vi "OrderDeviceList.vi"(8 "error in (no error)":errorcluster, 11 "Device List In":refnum<class "Device.lvclass">[](array[class])) -> (0 "error out":errorcluster, 2 "Changes Made":bool, 3 "Device List Out":refnum<class "Device.lvclass">[](array[class]))   [LabVIEW 2013]
uses:
  DeviceVIs/Device/Device.lvclass
  DeviceVIs/Pulseblaster/Pulseblaster.lvclass
  ColumnVIs/Column/Column.lvclass
  ColumnVIs/ModeCol/ModeCol.lvclass
  ColumnVIs/GroupCol/GroupCol.lvclass
  ColumnVIs/DigitalCol/DigitalCol.lvclass
  ColumnVIs/TriggerCol/TriggerCol.lvclass
  DeviceVIs/NI Card/NI Card.lvclass
  DeviceVIs/Slave_Pulseblaster/Slave_Pulseblaster.lvclass
panel:
  in  "Cancel Button":bool
  in  "OK Button":bool
  out "Master Name":string="Master Device"
  in  "Device Order":i32(listbox)
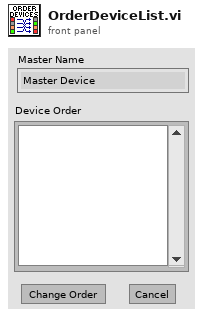
[diagram p1: front panel]
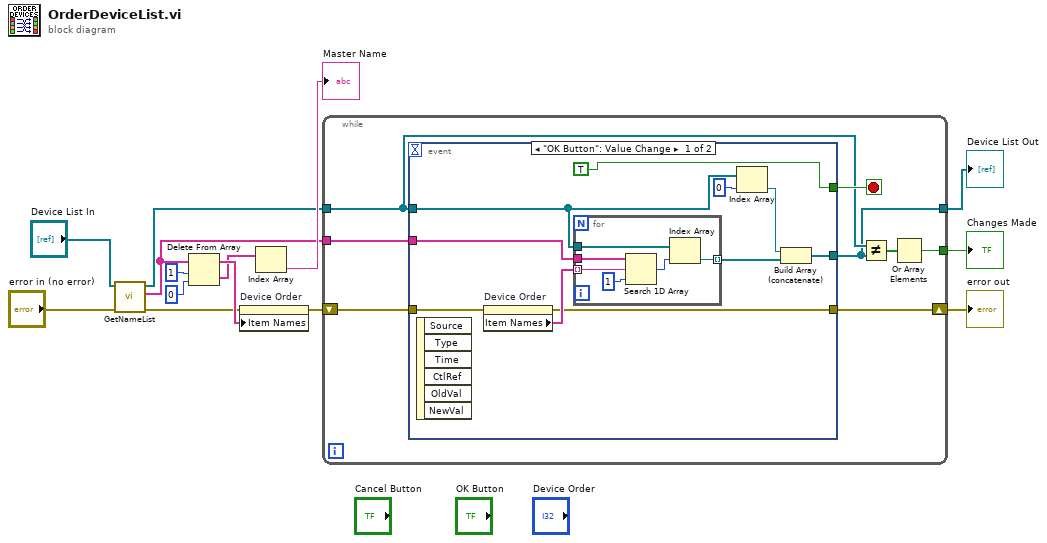
[diagram p0: block diagram]
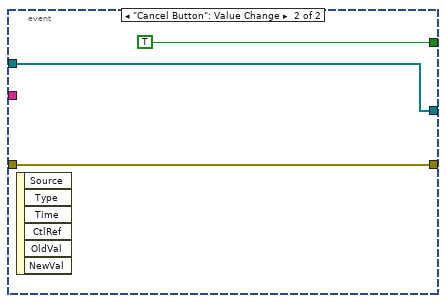
[diagram p2: hidden frame]
diagram:
  n1 = call "GetNameList.vi"("error in (no error)"="error in (no error)", "Devices"="Device List In") -> ("error out"=w6:errorcluster, "Names in use"=w9:string[], "Devices out"=w4:refnum<class "Device.lvclass">[])  [unwired: 7 in]
  n2 = Delete From Array(array=w9, length=1, index=0) -> (deleted portion=w11:string[], array with subset deleted=w13:string[])
  n3 = property on="Device Order" class="LstBox (strict)"(error in=w6, "Item Names"=w13) -> (error out=w5:errorcluster)  [unwired: 1 in, 1 out]
  n4 = Index Array(array=w11) -> (element=→"Master Name":string)  [unwired: 1 in]
  n5 = while {
    tunnel: w9 -> [w20]
    tunnel: [w19] -> w8
    shift-right: [w18] -> w1
    shift-left: w5 -> [w21]
    tunnel: w4 -> [w16]
    tunnel: [w15] -> w2
    stop <- w22 stop-if-true
    n6 = event shown="[0] \"OK Button\": Value Change" {
      selector: _ -> [_ _]
      dyn-events: _ -> [_ _]
      timeout: _ -> [_ _]
      tunnel: [TRUE TRUE] -> w22
      tunnel: w21 -> [w28 w40]
      tunnel: w20 -> [w29 _]
      tunnel: [w26 w39] -> w15
      tunnel: [w24 w40] -> w18
      tunnel: w16 -> [w23 w39]
      event "OK Button": Value Change {
        n7 = event-data() -> ()  [unwired: 1 in, 6 out]
        n8 = property on="Device Order" class="LstBox (strict)"(error in=w28) -> (error out=w24:errorcluster, "Item Names"=w30:string[])  [unwired: 1 in, 1 out]
        n9 = for {
          tunnel: w30 -> [w38] mode=indexing
          tunnel: w29 -> [w37]
          tunnel: [w34] -> w25 mode=indexing
          tunnel: w23 -> [w33]
          n10 = Search 1D Array(1D array=w37, element=w38, start index (0)=1) -> (index of element=w35:i32)
          n11 = Index Array(array=w33, index=w35) -> (element=w34:refnum<class "Device.lvclass">)
        }
        n12 = Index Array(array=w23, index=0) -> (element=w31:refnum<class "Device.lvclass">)
        n13 = Build Array (concatenate)(w31, w25) -> (w26:refnum<class "Device.lvclass">[])
      }
      event "Cancel Button": Value Change {
        n14 = event-data() -> ()  [unwired: 1 in, 6 out]
      }
    }
    n15 = Not Equal?(x=w16, y=w15) -> (x != y?=w17:bool[])
    n16 = Or Array Elements(Boolean array=w17) -> (logical OR=w19:bool)
  }
  "Device List Out" <- w2
  "Changes Made" <- w8
  "error out" <- w1
